vi "Write XML Document.lvclass.vi"(8 "error in":errorcluster, 10 "XML Document.lvclass":refnum<class "XML Document.lvclass">, 11 "XML Editor GUI in":refnum<class "XML Editor GUI.lvclass">) -> (0 "error out":errorcluster, 3 "XML Editor GUI out":refnum<class "XML Editor GUI.lvclass">)   [LabVIEW 2014, in "XML Editor GUI.lvclass"]
uses:
  XML Editor GUI.lvclass
  XML Document_class/XML Document.lvclass
  XML Editor GUI.lvclass/XML Editor GUI.ctl
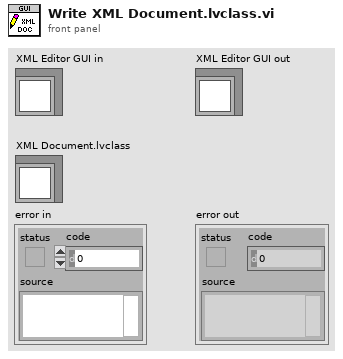
[diagram p1: front panel]
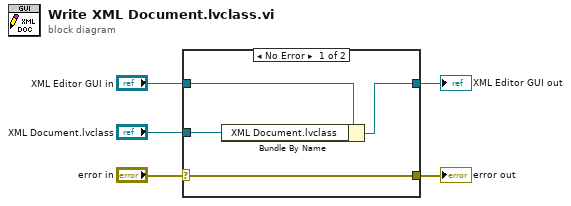
[diagram p0: block diagram]
diagram:
  n1 = case shown="No Error" "error in" {
    selector: "error in" -> [w9 w10]
    tunnel: [w9 w10] -> w4
    tunnel: [w7 w11] -> w2
    tunnel: "XML Editor GUI in" -> [w8 w11]
    tunnel: "XML Document.lvclass" -> [w6 _]
    frame No Error {
      n2 = Bundle By Name(cluster=w8, "XML Document.lvclass"=w6) -> (w7:refnum<class "XML Editor GUI.lvclass">)
    }
    frame Error {
    }
  }
  "error out" <- w4
  "XML Editor GUI out" <- w2
